vi "write_y.vi"(8 "error in (no error)":errorcluster, 10 "y":dbl[][](array[numeric]), 11 "MultiTaskLassoCV in":refnum<class "MultiTaskLassoCV.lvclass">) -> (0 "error out":errorcluster, 3 "MultiTaskLassoCV out":refnum<class "MultiTaskLassoCV.lvclass">)   [LabVIEW 2020, in "MultiTaskLassoCV.lvclass"]
uses:
  MultiTaskLassoCV.lvclass
  MultiTaskLassoCV.lvclass/MultiTaskLassoCV.ctl
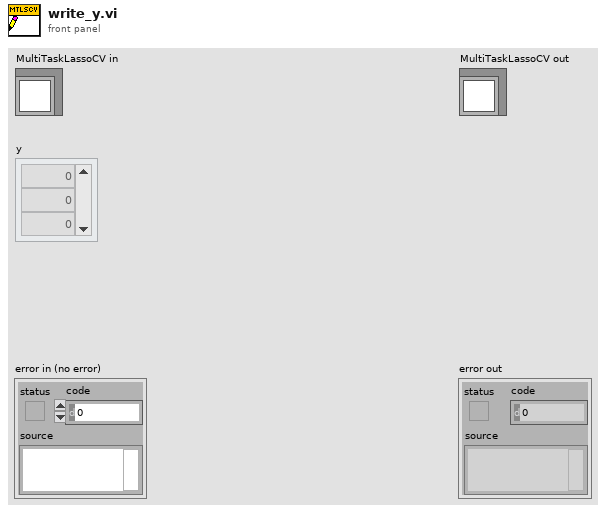
[diagram p1: front panel]
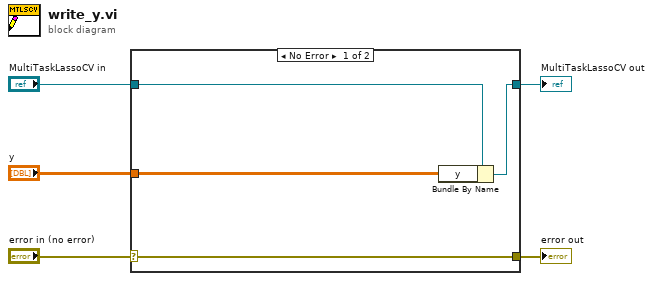
[diagram p0: block diagram]
diagram:
  n1 = case shown="No Error" "error in (no error)" {
    selector: "error in (no error)" -> [w9 w10]
    tunnel: [w9 w10] -> w4
    tunnel: [w7 w11] -> w2
    tunnel: "MultiTaskLassoCV in" -> [w8 w11]
    tunnel: "y" -> [w6 _]
    frame No Error {
      n2 = Bundle By Name(cluster=w8, "y"=w6) -> (w7:refnum<class "MultiTaskLassoCV.lvclass">)
    }
    frame Error {
    }
  }
  "error out" <- w4
  "MultiTaskLassoCV out" <- w2
